vi "read TBM configuration.vi"(8 "error in":errorcluster, 11 "Tag Bus Web Interface editor node in":refnum<class "Tag Bus Web Interface editor node.lvclass">) -> (0 "error out":errorcluster, 2 "TBM configuration out":refnum<class "TBM configuration.lvclass">, 3 "Tag Bus Web Interface editor node out":refnum<class "Tag Bus Web Interface editor node.lvclass">)   [LabVIEW 2013, in "Tag Bus Web Interface editor node.lvclass"]
uses:
  Tag Bus Web Interface editor node.lvclass
  <vilib>/NI/Tag Bus Module Framework/root configuration/TBM configuration.lvclass
  Tag Bus Web Interface editor node.lvclass/Tag Bus Web Interface editor node.ctl
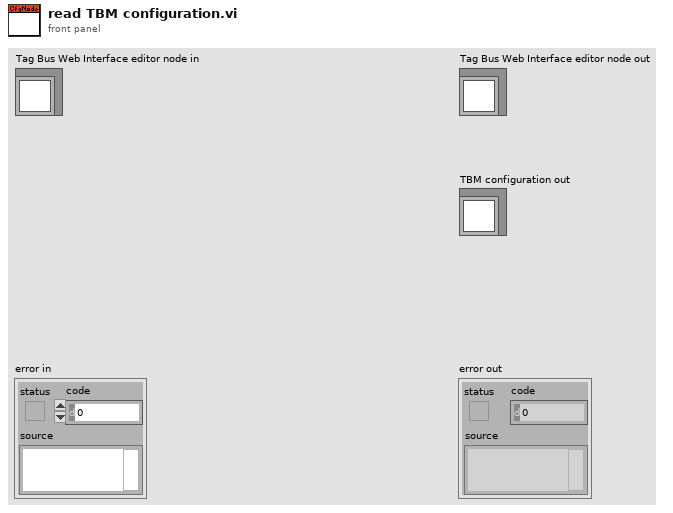
[diagram p1: front panel]
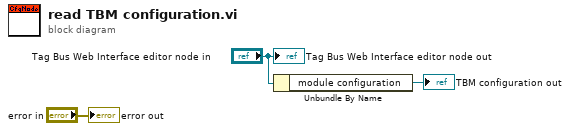
[diagram p0: block diagram]
diagram:
  n1 = Unbundle By Name("Tag Bus Web Interface editor node in") -> ("module configuration"=→"TBM configuration out":refnum<class "Tag Bus Web Interface configuration.lvclass">)
  "error out" <- "error in"
  "Tag Bus Web Interface editor node out" <- "Tag Bus Web Interface editor node in"
